vi "readAvailable.vi"(8 "error in (no error)":errorcluster, 11 "SerialSimulator in":refnum<class "SerialSimulator.lvclass">) -> (0 "error out":errorcluster, 2 "stringRead":string, 3 "SerialSimulator out":refnum<class "SerialSimulator.lvclass">)   [LabVIEW 2015, in "SerialProtocols.lvlib" / "SerialSimulator.lvclass"]
uses:
  <userlib>/Common/SerialProtocols/SerialProtocol/SerialSimulator/SerialSimulator.lvclass
  <userlib>/Common/SerialProtocols/SerialProtocol/SerialSimulator/SerialSimulator.lvclass/SerialSimulator.ctl
  <userlib>/Common/Simulators/SimulateSerialData/SimulateSerialData.lvclass
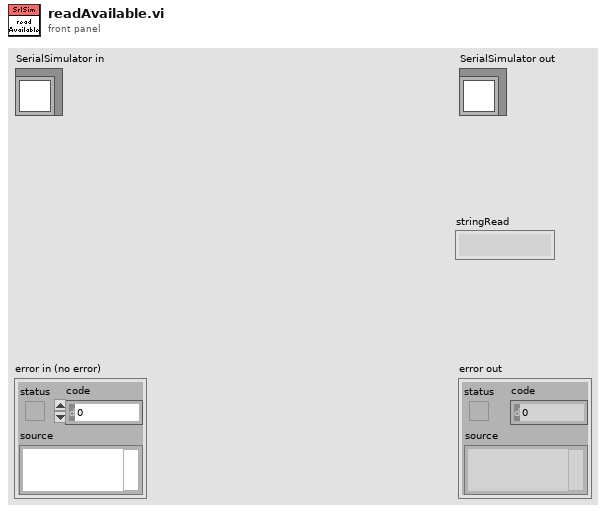
[diagram p1: front panel]
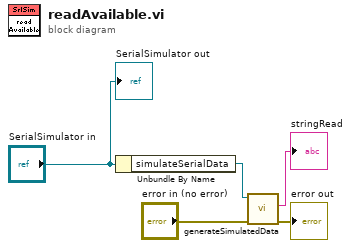
[diagram p0: block diagram]
diagram:
  n1 = Unbundle By Name("SerialSimulator in") -> ("simulateSerialData"=w4:refnum<class "SimulateSerialData.lvclass">)
  n2 = call-dynamic "generateSimulatedData.vi"("error in (no error)"="error in (no error)", "SimulateSerialData in"=w4) -> ("error out"=→"error out":errorcluster, "stringRead"=→"stringRead":string)  [unwired: 7 in, 1 out]
  "SerialSimulator out" <- "SerialSimulator in"
